vi "simula cmecc.vi"(0 "RPM":dbl format="%#_13g", 1 "C":dbl format="%#_13g", 2 "String":string="CARICO", 3 "V":dbl format="%#_13g") -> (12 "RPM":dbl, 14 "cosfi":dbl, 15 "C[nm]":dbl, 16 "I[A]":dbl, 17 "Pin kw":dbl, 18 "Pout kw":dbl, 19 "eff%":dbl)   [LabVIEW 2019]
uses:
  <vilib>/gmath/NI_Gmath.lvlib
panel:
  in  "VUOTO":string[][](array[string])=[["n°Acq", "Freq [Hz]", "RPM", "Vtr [V]", "Vts [V]", "Vsr [V]", "It [A]", "Ir [A]", "Is [A]", "Vmean [V]", "Imean [A]", "Irec [A]", "Irec/In", "CosFi", "P in [kW]", "P out [kW]", "Eff [%]", "T [Nm]", "Trec [Nm]", "Trec/Cn", "Slip [%]", "R1 [Ohm]", "dT1 [°C]", "Tamb [°C]", "TC1 [°C]", "TC2 [°C]", "TC3 [°C]", "Time [min]", "Date\\time"], ["1", "49.99", "2990", "441.34", "414.63", "442.09", "1.90", "1.98", "2.04", "441.72", "1.97", "1.78", "0.76", "0.125", "0.189", "0.000", "0.00", "0.01", "0.01", "0.00", "100.00", "14.20449", "0.79", "21.8", "32.9", "30.7", "28.8", "1.373", "24/05/2017 16:33:41"], ["2", "50.00", "2990", "399.24", "374.56", "401.38", "1.14", "1.25", "1.30", "400.31", "1.22", "1.22", "0.52", "0.142", "0.121", "0.000", "0.00", "0.01", "0.01", "0.00", "100.00", "14.24889", "1.58", "21.9", "32.5", "29.7", "28.2", "1.890", "24/05/2017 16:34:12"], ["3", "50.01", "2990", "377.89", "353.26", "380.50", "0.90", "1.02", "1.07", "379.20", "0.99", "1.04", "0.44", "0.161", "0.104", "0.000", "0.00", "0.01", "0.01", "0.00", "100.00", "14.19922", "0.69", "21.8", "32.1", "29.2", "27.9", "2.373", "24/05/2017 16:34:41"], ["4", "50.02", "2990", "359.59", "333.88", "361.83", "0.77", "0.89", "0.91", "360.71", "0.84", "0.93", "0.39", "0.182", "0.095", "0.000", "0.00", "0.01", "0.01", "0.00", "100.00", "14.12952", "-0.59", "21.9", "31.9", "28.8", "27.7", "2.866", "24/05/2017 16:35:11"], ["5", "49.98", "2990", "239.37", "220.27", "242.66", "0.39", "0.51", "0.52", "241.01", "0.46", "0.76", "0.32", "0.340", "0.065", "0.000", "0.00", "0.01", "0.02", "0.00", "100.00", "14.03546", "-2.31", "21.9", "31.5", "28.6", "27.5", "3.440", "24/05/2017 16:35:45"], ["6", "49.99", "2990", "199.14", "180.73", "202.29", "0.33", "0.44", "0.44", "200.72", "0.38", "0.76", "0.32", "0.440", "0.059", "0.000", "0.00", "0.01", "0.02", "0.01", "100.00", "13.96122", "-3.66", "21.9", "31.3", "28.4", "27.4", "3.890", "24/05/2017 16:36:12"], ["7", "49.99", "2990", "159.38", "140.24", "162.50", "0.27", "0.41", "0.37", "160.94", "0.32", "0.81", "0.34", "0.599", "0.054", "0.000", "0.00", "0.01", "0.04", "0.01", "100.00", "13.90466", "-4.68", "21.9", "31.0", "28.2", "27.2", "4.256", "24/05/2017 16:36:34"], ["8", "49.99", "2990", "120.04", "101.13", "122.43", "0.28", "0.38", "0.34", "121.23", "0.31", "1.03", "0.43", "0.790", "0.052", "0.000", "0.00", "0.01", "0.06", "0.02", "100.00", "13.84049", "-5.84", "21.9", "30.7", "27.9", "27.0", "4.703", "24/05/2017 16:37:01"]]
  in  "CARICO":string[][](array[string])=[["n°Acq", "Freq [Hz]", "RPM", "Vtr [V]", "Vts [V]", "Vsr [V]", "It [A]", "Ir [A]", "Is [A]", "Vmean [V]", "Imean [A]", "Irec [A]", "Irec/In", "CosFi", "P in [kW]", "P out [kW]", "Eff [%]", "T [Nm]", "Trec [Nm]", "Trec/Cn", "Slip [%]", "R1 [Ohm]", "dT1 [°C]", "Tamb [°C]", "TC1 [°C]", "TC2 [°C]", "TC3 [°C]", "Time [min]", "Date\\time"], ["1", "50.01", "2806.2", "400.30", "376.15", "401.45", "2.86", "2.99", "2.95", "400.87", "2.90", "2.89", "1.23", "0.880", "1.771", "1.372", "77.48", "4.67", "4.65", "1.27", "6.47", "14.78061", "8.97", "21.9", "33.2", "30.2", "28.9", "1.737", "24/05/2017 16:26:19"], ["2", "50.00", "2828.6", "400.27", "376.11", "401.72", "2.57", "2.72", "2.67", "400.99", "2.62", "2.62", "1.11", "0.870", "1.585", "1.246", "78.58", "4.21", "4.18", "1.15", "5.71", "15.05714", "13.92", "21.9", "33.0", "29.6", "28.6", "2.673", "24/05/2017 16:27:15"], ["3", "50.00", "2863.3", "399.24", "375.18", "400.70", "2.18", "2.32", "2.28", "399.97", "2.23", "2.23", "0.95", "0.843", "1.303", "1.043", "80.03", "3.48", "3.48", "0.95", "4.56", "15.05270", "13.85", "21.9", "32.9", "29.3", "28.6", "3.903", "24/05/2017 16:28:29"], ["4", "49.99", "2898.6", "398.36", "374.57", "400.21", "1.78", "1.93", "1.89", "399.29", "1.84", "1.84", "0.78", "0.788", "1.002", "0.808", "80.72", "2.66", "2.67", "0.73", "3.36", "14.99414", "12.80", "21.9", "32.9", "29.4", "28.5", "4.370", "24/05/2017 16:28:57"], ["5", "50.00", "2935.4", "397.64", "373.91", "399.71", "1.41", "1.56", "1.55", "398.67", "1.48", "1.48", "0.63", "0.667", "0.681", "0.535", "78.58", "1.74", "1.75", "0.48", "2.15", "14.88601", "10.84", "21.9", "32.8", "29.2", "28.4", "4.823", "24/05/2017 16:29:24"], ["6", "50.00", "2967.6", "398.04", "373.91", "400.09", "1.18", "1.33", "1.33", "399.06", "1.26", "1.26", "0.53", "0.446", "0.388", "0.267", "68.91", "0.86", "0.86", "0.24", "1.08", "14.75175", "8.44", "21.9", "32.8", "29.2", "28.3", "5.307", "24/05/2017 16:29:53"]]
  in  "CMECC":string[][](array[string])=[["n°Acq", "Freq [Hz]", "RPM", "Vtr [V]", "Vts [V]", "Vsr [V]", "It [A]", "Ir [A]", "Is [A]", "Vmean [V]", "Imean [A]", "Irec [A]", "Irec/In", "CosFi", "P in [kW]", "P out [kW]", "Eff [%]", "T [Nm]", "Trec [Nm]", "Trec/Cn", "Slip [%]", "R1 [Ohm]", "dT1 [°C]", "Tamb [°C]", "TC1 [°C]", "TC2 [°C]", "TC3 [°C]", "Time [min]", "Date\\time", "", "", "", ""], ["0", "49,8", "3010", "400", "377", "400", "0,8", "0,4", "0,7", "400", "0,85", "", "", "", "0,3", "0", "", "0", "", "", "", "", "", "", "", "", "", "", "", "", "", "", ""], ["1", "49.98", "2948.1", "399.34", "377.38", "401.04", "1.36", "1.49", "1.48", "400.19", "1.42", "1.42", "0.60", "0.608", "0.599", "0.455", "75.96", "1.47", "1.47", "0.40", "1.69", "-1.00000", "0.00", "22.3", "30.3", "28.4", "27.3", "0.977", "25/05/2017 14:23:00", "", "", "", ""], ["2", "49.98", "2902.9", "398.17", "375.99", "399.91", "1.72", "1.85", "1.82", "399.04", "1.77", "1.77", "0.75", "0.766", "0.937", "0.810", "86.44", "2.66", "2.68", "0.73", "3.20", "-1.00000", "0.00", "22.3", "30.3", "28.4", "27.3", "0.989", "25/05/2017 14:23:00", "", "", "", ""], ["3", "49.98", "2853.7", "397.65", "376.18", "399.71", "2.30", "2.47", "2.43", "398.68", "2.37", "2.37", "1.01", "0.854", "1.396", "1.153", "82.60", "3.86", "3.88", "1.06", "4.84", "-1.00000", "0.00", "22.3", "30.3", "28.4", "27.3", "1.001", "25/05/2017 14:23:01", "", "", "", ""], ["4", "49.99", "2803.6", "396.44", "374.24", "398.18", "2.88", "3.01", "3.00", "397.31", "2.94", "2.96", "1.25", "0.882", "1.784", "1.427", "79.99", "4.86", "4.93", "1.35", "6.52", "-1.00000", "0.00", "22.3", "30.2", "28.4", "27.2", "1.014", "25/05/2017 14:23:02", "", "", "", ""], ["5", "49.99", "2759.2", "397.71", "375.43", "399.21", "3.46", "3.58", "3.56", "398.46", "3.51", "3.52", "1.49", "0.891", "2.157", "1.644", "76.22", "5.69", "5.73", "1.57", "8.01", "-1.00000", "0.00", "22.3", "30.2", "28.4", "27.2", "1.027", "25/05/2017 14:23:03", "", "", "", ""], ["6", "49.99", "2710.3", "395.68", "373.27", "397.27", "3.98", "4.10", "4.08", "396.47", "4.03", "4.07", "1.72", "0.895", "2.479", "1.807", "72.88", "6.37", "6.48", "1.78", "9.64", "-1.00000", "0.00", "22.3", "30.2", "28.4", "27.2", "1.040", "25/05/2017 14:23:03", "", "", "", ""], ["7", "49.92", "2666.1", "396.88", "375.28", "398.43", "4.44", "4.54", "4.54", "397.66", "4.49", "4.51", "1.91", "0.894", "2.765", "1.942", "70.23", "6.96", "7.04", "1.93", "10.99", "-1.00000", "0.00", "22.3", "30.2", "28.3", "27.2", "1.052", "25/05/2017 14:23:04", "", "", "", ""], ["8", "49.99", "2623.2", "395.30", "373.16", "396.73", "4.85", "4.93", "4.94", "396.01", "4.89", "4.94", "2.09", "0.894", "3.001", "2.029", "67.61", "7.39", "7.54", "2.06", "12.54", "-1.00000", "0.00", "22.3", "30.2", "28.3", "27.2", "1.062", "25/05/2017 14:23:05", "", "", "", ""], ["9", "49.99", "2560.8", "394.56", "372.80", "396.07", "5.43", "5.52", "5.52", "395.31", "5.47", "5.54", "2.35", "0.892", "3.344", "2.184", "65.30", "8.14", "8.34", "2.28", "14.63", "-1.00000", "0.00", "22.3", "30.2", "28.3", "27.2", "1.073", "25/05/2017 14:23:05", "", "", "", ""], ["10", "49.99", "2490.5", "400.92", "378.49", "402.07", "6.10", "6.19", "6.16", "401.50", "6.13", "6.11", "2.59", "0.888", "3.787", "2.319", "61.25", "8.89", "8.83", "2.42", "16.96", "-1.00000", "0.00", "22.3", "30.2", "28.3", "27.2", "1.083", "25/05/2017 14:23:06", "", "", "", ""], ["11", "49.99", "2409.2", "400.46", "378.67", "402.05", "6.79", "6.88", "6.88", "401.25", "6.84", "6.81", "2.89", "0.884", "4.199", "2.342", "55.79", "9.28", "9.23", "2.53", "19.68", "-1.00000", "0.00", "22.3", "30.2", "28.3", "27.2", "1.093", "25/05/2017 14:23:07", "", "", "", ""], ["12", "49.99", "2338.6", "400.74", "377.60", "402.36", "7.33", "7.43", "7.42", "401.55", "7.37", "7.35", "3.11", "0.879", "4.508", "2.357", "52.29", "9.63", "9.55", "2.62", "22.03", "-1.00000", "0.00", "22.3", "30.2", "28.3", "27.2", "1.103", "25/05/2017 14:23:07", "", "", "", ""], ["13", "49.98", "2266.1", "400.56", "376.81", "401.95", "7.83", "7.93", "7.90", "401.25", "7.87", "7.84", "3.32", "0.874", "4.781", "2.338", "48.91", "9.85", "9.79", "2.68", "24.44", "-1.00000", "0.00", "22.3", "30.2", "28.3", "27.2", "1.113", "25/05/2017 14:23:08", "", "", "", ""], ["14", "50.00", "2194.0", "400.26", "377.09", "401.37", "8.28", "8.38", "8.35", "400.82", "8.31", "8.29", "3.51", "0.870", "5.018", "2.298", "45.79", "10.00", "9.96", "2.73", "26.87", "-1.00000", "0.00", "22.3", "30.2", "28.3", "27.2", "1.124", "25/05/2017 14:23:08", "", "", "", ""], ["15", "50.00", "2126.8", "399.39", "376.25", "401.11", "8.66", "8.76", "8.73", "400.25", "8.69", "8.69", "3.68", "0.866", "5.217", "2.245", "43.03", "10.08", "10.07", "2.76", "29.10", "-1.00000", "0.00", "22.3", "30.2", "28.3", "27.2", "1.134", "25/05/2017 14:23:09", "", "", "", ""], ["16", "49.99", "2052.7", "401.77", "378.90", "403.07", "9.02", "9.14", "9.10", "402.42", "9.06", "9.01", "3.82", "0.863", "5.449", "2.181", "40.02", "10.15", "10.02", "2.75", "31.56", "-1.00000", "0.00", "22.3", "30.2", "28.3", "27.2", "1.144", "25/05/2017 14:23:10", "", "", "", ""], ["17", "49.98", "1980.2", "397.93", "375.13", "399.39", "9.34", "9.45", "9.40", "398.66", "9.37", "9.41", "3.99", "0.858", "5.553", "2.075", "37.36", "10.00", "10.07", "2.76", "33.97", "-1.00000", "0.00", "22.3", "30.3", "28.3", "27.2", "1.154", "25/05/2017 14:23:10", "", "", "", ""], ["18", "49.98", "1916.4", "398.56", "374.54", "399.91", "9.63", "9.74", "9.70", "399.23", "9.67", "9.69", "4.10", "0.855", "5.713", "2.026", "35.46", "10.09", "10.13", "2.78", "36.09", "-1.00000", "0.00", "22.3", "30.3", "28.3", "27.2", "1.164", "25/05/2017 14:23:11", "", "", "", ""], ["19", "49.99", "1844.1", "398.95", "376.55", "400.02", "9.91", "10.04", "10.00", "399.48", "9.96", "9.97", "4.22", "0.851", "5.865", "1.925", "32.83", "9.97", "10.00", "2.74", "38.51", "-1.00000", "0.00", "22.3", "30.3", "28.3", "27.2", "1.174", "25/05/2017 14:23:11", "", "", "", ""], ["20", "49.98", "1771.5", "397.82", "375.33", "398.67", "10.15", "10.27", "10.21", "398.25", "10.18", "10.22", "4.33", "0.848", "5.955", "1.814", "30.46", "9.78", "9.86", "2.70", "40.93", "-1.00000", "0.00", "22.2", "30.3", "28.3", "27.3", "1.185", "25/05/2017 14:23:12", "", "", "", ""], ["21", "49.98", "1706.2", "397.07", "374.33", "397.98", "10.37", "10.46", "10.40", "397.53", "10.39", "10.45", "4.43", "0.845", "6.044", "1.733", "28.68", "9.70", "9.82", "2.69", "43.11", "-1.00000", "0.00", "22.2", "30.3", "28.3", "27.3", "1.195", "25/05/2017 14:23:13", "", "", "", ""], ["22", "49.99", "1634.2", "397.30", "374.02", "398.72", "10.57", "10.68", "10.64", "398.01", "10.61", "10.66", "4.52", "0.843", "6.163", "1.652", "26.80", "9.65", "9.75", "2.67", "45.52", "-1.00000", "0.00", "22.2", "30.3", "28.3", "27.3", "1.205", "25/05/2017 14:23:13", "", "", "", ""], ["23", "49.99", "1552.9", "396.22", "373.07", "397.11", "10.79", "10.88", "10.85", "396.67", "10.82", "10.91", "4.62", "0.839", "6.236", "1.530", "24.53", "9.41", "9.57", "2.62", "48.23", "-1.00000", "0.00", "22.2", "30.3", "28.3", "27.3", "1.215", "25/05/2017 14:23:14", "", "", "", ""], ["24", "49.99", "1478.5", "398.04", "375.15", "398.88", "11.02", "11.12", "11.05", "398.46", "11.04", "11.08", "4.69", "0.838", "6.378", "1.443", "22.62", "9.32", "9.39", "2.57", "50.70", "-1.00000", "0.00", "22.3", "30.5", "28.3", "27.4", "1.225", "25/05/2017 14:23:14", "", "", "", ""], ["25", "49.98", "1409.6", "396.79", "373.74", "398.12", "11.15", "11.25", "11.21", "397.46", "11.18", "11.26", "4.77", "0.835", "6.431", "1.350", "20.99", "9.14", "9.26", "2.54", "53.00", "-1.00000", "0.00", "22.3", "30.5", "28.3", "27.4", "1.235", "25/05/2017 14:23:15", "", "", "", ""], ["26", "49.98", "1346.7", "396.48", "373.50", "397.29", "11.28", "11.39", "11.34", "396.89", "11.31", "11.40", "4.83", "0.833", "6.474", "1.263", "19.50", "8.95", "9.09", "2.49", "55.09", "-1.00000", "0.00", "22.3", "30.5", "28.3", "27.4", "1.246", "25/05/2017 14:23:16", "", "", "", ""], ["27", "49.99", "1265.5", "396.37", "373.49", "396.93", "11.37", "11.48", "11.41", "396.65", "11.39", "11.49", "4.87", "0.832", "6.510", "1.151", "17.69", "8.69", "8.84", "2.42", "57.81", "-1.00000", "0.00", "22.3", "30.6", "28.3", "27.5", "1.256", "25/05/2017 14:23:16", "", "", "", ""], ["28", "49.98", "1212.3", "400.93", "377.63", "401.91", "11.64", "11.72", "11.68", "401.42", "11.66", "11.62", "4.92", "0.832", "6.741", "1.138", "16.89", "8.97", "8.90", "2.44", "59.57", "-1.00000", "0.00", "22.3", "30.6", "28.3", "27.5", "1.266", "25/05/2017 14:23:17", "", "", "", ""], ["29", "49.99", "1137.2", "403.35", "380.25", "404.47", "11.91", "11.98", "11.88", "403.91", "11.90", "11.78", "4.99", "0.830", "6.908", "1.062", "15.37", "8.92", "8.75", "2.40", "62.08", "-1.00000", "0.00", "22.3", "30.6", "28.3", "27.5", "1.276", "25/05/2017 14:23:18", "", "", "", ""], ["30", "49.98", "1058.9", "402.43", "378.57", "403.46", "11.93", "12.03", "12.00", "402.94", "11.97", "11.88", "5.03", "0.829", "6.923", "0.946", "13.66", "8.53", "8.40", "2.30", "64.69", "-1.00000", "0.00", "22.3", "30.6", "28.3", "27.5", "1.286", "25/05/2017 14:23:18", "", "", "", ""], ["31", "49.97", "986.7", "401.35", "378.20", "402.45", "12.00", "12.07", "12.05", "401.90", "12.03", "11.97", "5.07", "0.827", "6.928", "0.859", "12.40", "8.31", "8.24", "2.26", "67.09", "-1.00000", "0.00", "22.3", "30.7", "28.4", "27.6", "1.297", "25/05/2017 14:23:19", "", "", "", ""], ["32", "49.99", "920.0", "402.00", "378.51", "403.04", "12.08", "12.17", "12.13", "402.52", "12.11", "12.03", "5.10", "0.827", "6.975", "0.791", "11.34", "8.21", "8.11", "2.22", "69.33", "-1.00000", "0.00", "22.3", "30.7", "28.4", "27.6", "1.307", "25/05/2017 14:23:19", "", "", "", ""], ["33", "49.98", "850.8", "401.64", "378.11", "402.78", "12.17", "12.25", "12.22", "402.21", "12.19", "12.13", "5.14", "0.826", "7.013", "0.705", "10.06", "7.92", "7.83", "2.14", "71.63", "-1.00000", "0.00", "22.3", "30.7", "28.4", "27.6", "1.317", "25/05/2017 14:23:20", "", "", "", ""], ["34", "49.97", "777.8", "400.86", "378.12", "402.49", "12.19", "12.27", "12.23", "401.67", "12.21", "12.16", "5.15", "0.825", "7.007", "0.640", "9.13", "7.85", "7.79", "2.13", "74.06", "-1.00000", "0.00", "22.3", "30.9", "28.5", "27.8", "1.327", "25/05/2017 14:23:21", "", "", "", ""], ["35", "49.97", "705.5", "400.85", "378.16", "403.38", "12.26", "12.37", "12.34", "402.12", "12.30", "12.23", "5.18", "0.825", "7.069", "0.562", "7.96", "7.61", "7.53", "2.06", "76.47", "-1.00000", "0.00", "22.3", "30.9", "28.5", "27.8", "1.337", "25/05/2017 14:23:21", "", "", "", ""], ["36", "49.98", "637.0", "401.49", "378.85", "403.76", "12.34", "12.45", "12.41", "402.62", "12.37", "12.29", "5.21", "0.824", "7.112", "0.490", "6.88", "7.34", "7.24", "1.98", "78.76", "-1.00000", "0.00", "22.3", "30.9", "28.5", "27.8", "1.347", "25/05/2017 14:23:22", "", "", "", ""], ["37", "49.99", "578.9", "401.68", "378.71", "403.39", "12.34", "12.46", "12.42", "402.53", "12.38", "12.30", "5.21", "0.824", "7.109", "0.443", "6.23", "7.30", "7.21", "1.98", "80.70", "-1.00000", "0.00", "22.3", "30.9", "28.5", "27.8", "1.358", "25/05/2017 14:23:22", "", "", "", ""], ["38", "49.98", "489.3", "399.20", "375.75", "400.56", "12.30", "12.39", "12.34", "399.88", "12.32", "12.32", "5.22", "0.822", "7.009", "0.359", "5.13", "7.01", "7.02", "1.92", "83.69", "-1.00000", "0.00", "22.3", "31.0", "28.7", "28.0", "1.368", "25/05/2017 14:23:23", "", "", "", ""], ["39", "49.98", "436.2", "396.67", "374.25", "397.73", "12.21", "12.28", "12.26", "397.20", "12.24", "12.33", "5.22", "0.822", "6.921", "0.315", "4.55", "6.90", "7.00", "1.92", "85.45", "-1.00000", "0.00", "22.3", "31.0", "28.7", "28.0", "1.378", "25/05/2017 14:23:24", "", "", "", ""], ["40", "50.02", "372.9", "398.90", "376.64", "399.52", "12.35", "12.37", "12.31", "399.21", "12.33", "12.35", "5.23", "0.823", "7.013", "0.274", "3.91", "7.02", "7.04", "1.93", "87.58", "-1.00000", "0.00", "22.3", "31.0", "28.7", "28.0", "1.388", "25/05/2017 14:23:24", "", "", "", ""], ["41", "49.99", "298.8", "399.29", "376.66", "399.94", "12.33", "12.41", "12.37", "399.62", "12.35", "12.36", "5.24", "0.821", "7.018", "0.222", "3.16", "7.09", "7.10", "1.95", "90.04", "-1.00000", "0.00", "22.3", "31.0", "28.7", "28.0", "1.399", "25/05/2017 14:23:25", "", "", "", ""], ["42", "49.97", "230.7", "398.30", "375.72", "399.25", "12.32", "12.37", "12.36", "398.78", "12.34", "12.38", "5.24", "0.821", "7.001", "0.173", "2.47", "7.15", "7.19", "1.97", "92.30", "-1.00000", "0.00", "22.3", "31.3", "28.8", "28.3", "1.409", "25/05/2017 14:23:25", "", "", "", ""], ["43", "49.98", "187.8", "399.13", "376.39", "399.68", "12.31", "12.37", "12.36", "399.41", "12.34", "12.35", "5.23", "0.822", "7.011", "0.152", "2.17", "7.75", "7.77", "2.13", "93.74", "-1.00000", "0.00", "22.3", "31.3", "28.8", "28.3", "1.419", "25/05/2017 14:23:26", "", "", "", ""], ["44", "50.00", "83.9", "399.74", "376.53", "400.38", "12.32", "12.37", "12.40", "400.06", "12.36", "12.36", "5.24", "0.823", "7.053", "0.069", "0.98", "7.88", "7.88", "2.16", "97.20", "-1.00000", "0.00", "22.3", "31.3", "28.8", "28.3", "1.429", "25/05/2017 14:23:27", "", "", "", ""], ["45", "49.97", "3,2", "399.16", "376.52", "400.07", "12.35", "12.43", "12.35", "399.62", "12.35", "12.36", "5.24", "0.824", "7.046", "0.003", "0.04", "7.87", "7.88", "2.16", "99.87", "-1.00000", "0.00", "22.3", "31.4", "29.0", "28.5", "1.440", "25/05/2017 14:23:27", "", "", "", ""]]
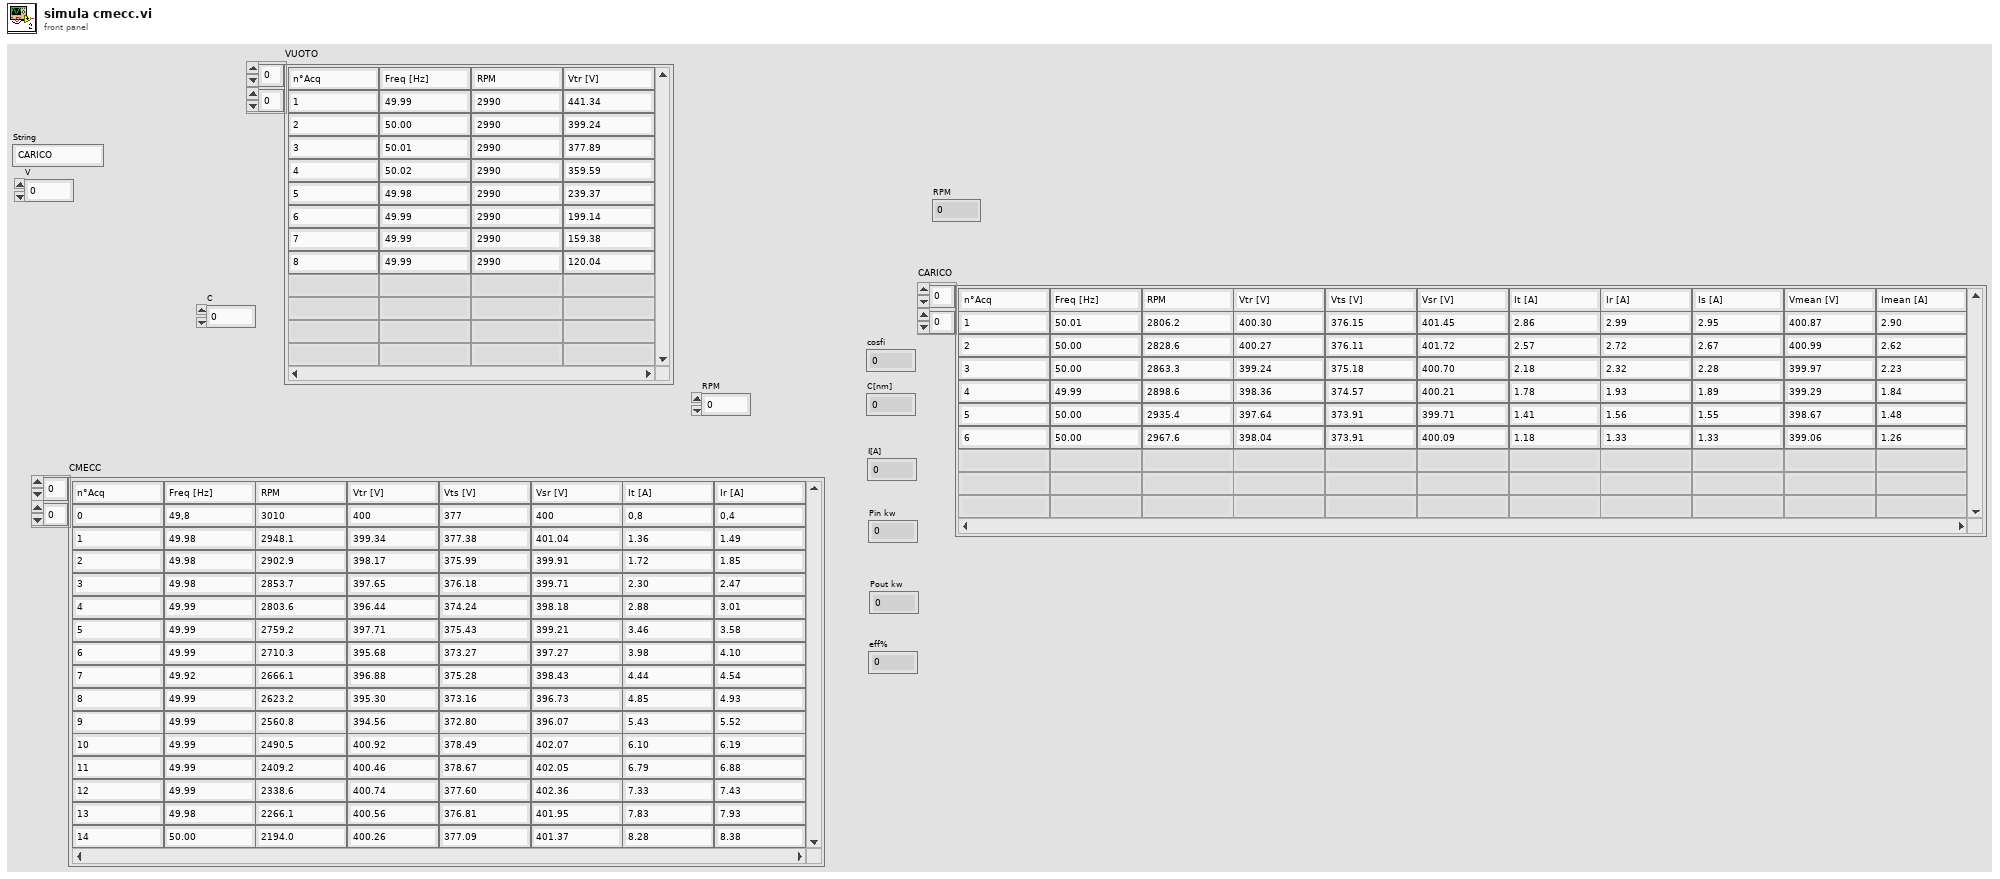
[diagram p1: front panel]
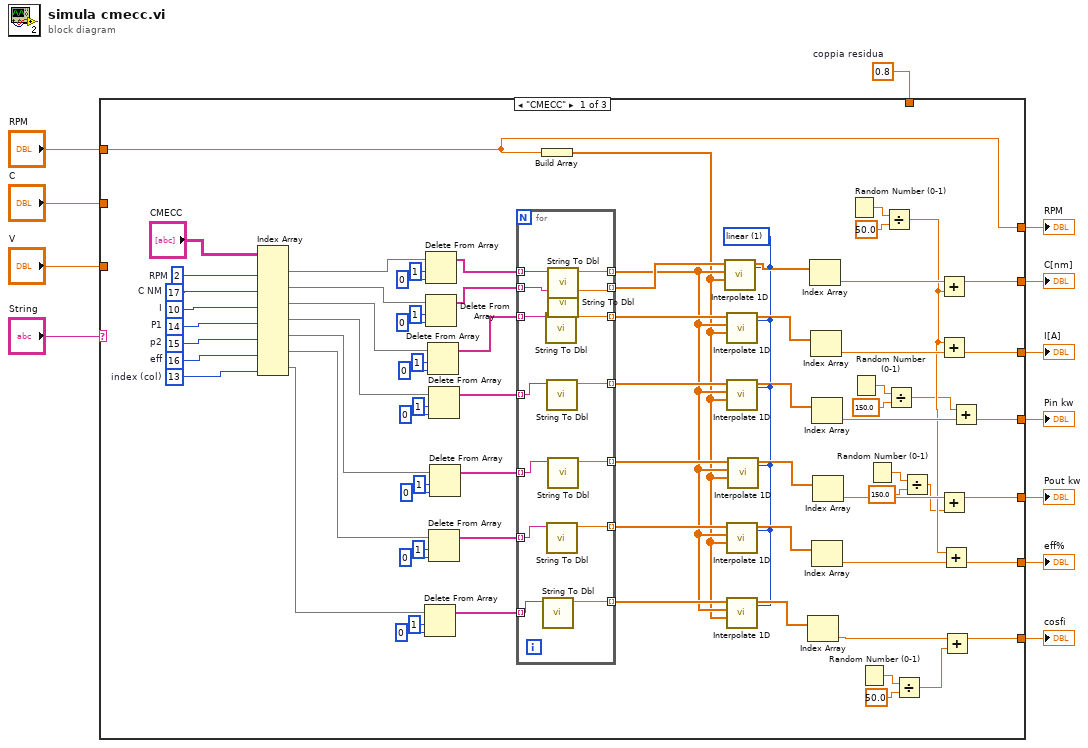
[diagram p0: block diagram]
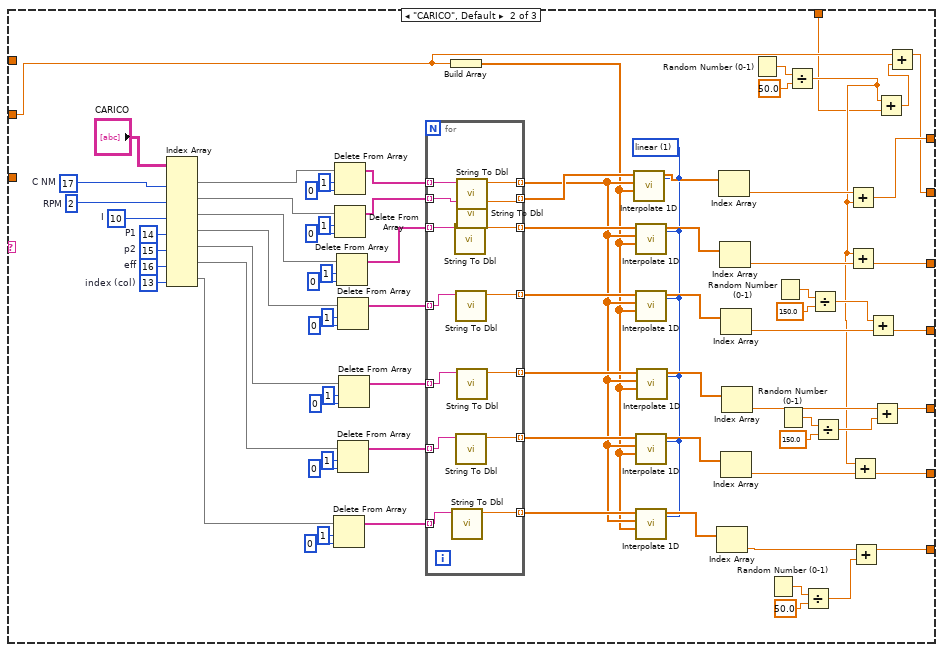
[diagram p2: hidden frame]
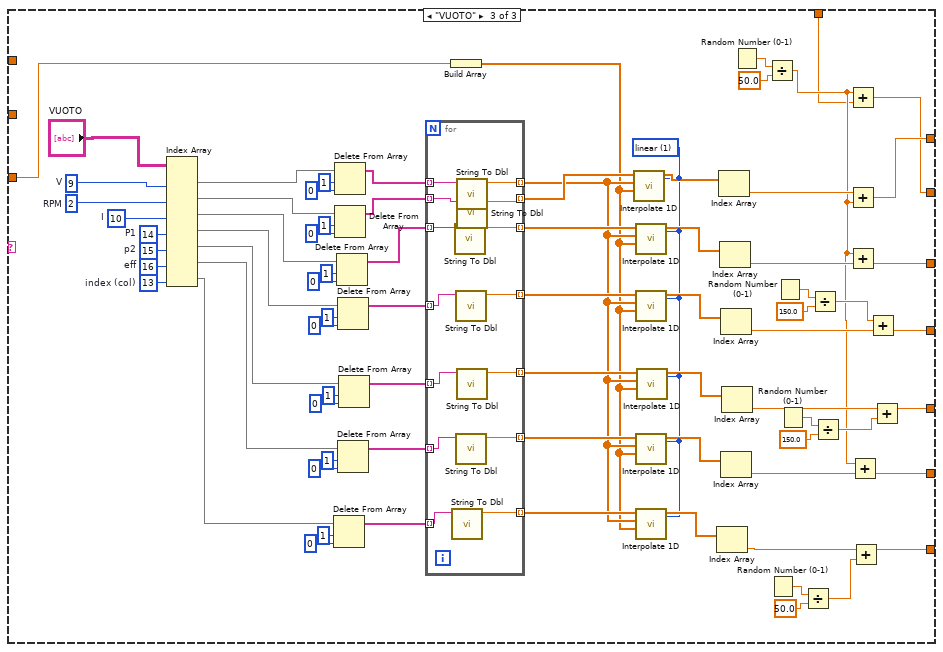
[diagram p3: hidden frame]
diagram:
  w1 = 0.8  # coppia residua
  n1 = case shown="\"CMECC\"" "String" {
    tunnel: [w29 w105 w196] -> w12
    tunnel: [w28 w127 w219] -> w11
    tunnel: [w27 w126 w218] -> w10
    tunnel: [w26 w125 w217] -> w9
    tunnel: [w25 w124 w216] -> w8
    tunnel: [w24 w123 w215] -> w7
    tunnel: "RPM" -> [w19 _ _]
    tunnel: "C" -> [_ w115 _]
    tunnel: [w19 w116 w209] -> w3
    tunnel: "V" -> [_ _ w201]
    tunnel: w1 -> [_ w103 w197]
    frame "CMECC" {
      w42 = 13  # index (col)
      w50 = 16  # eff
      w52 = 15  # p2
      w59 = 14  # P1
      w72 = 10  # I
      w32 = 1 items=["nearest", "linear", "spline", "cubic Hermite", "Lagrange"] ("method")
      w83 = 17  # C NM
      w87 = 2  # RPM
      n2 = Index Array(array="CMECC", index (col) #1=w87, index (col) #2=w83, index (col) #3=w72, index (col) #4=w59, index (col) #5=w52, index (col) #6=w50, index (col) #7=w42) -> (element #1=w82:string[], element #2=w76:string[], element #3=w71:string[], element #4=w61:string[], element #5=w51:string[], element #6=w43:string[], element #7=w36:string[])  [unwired: 7 in]
      n3 = Delete From Array(array=w36, length=1, index=0) -> (array with subset deleted=w41:string[])  [unwired: 1 out]
      n4 = Delete From Array(array=w82, length=1, index=0) -> (array with subset deleted=w81:string[])  [unwired: 1 out]
      n5 = Delete From Array(array=w76, length=1, index=0) -> (array with subset deleted=w75:string[])  [unwired: 1 out]
      n6 = Delete From Array(array=w71, length=1, index=0) -> (array with subset deleted=w70:string[])  [unwired: 1 out]
      n7 = Delete From Array(array=w61, length=1, index=0) -> (array with subset deleted=w60:string[])  [unwired: 1 out]
      n8 = Delete From Array(array=w43, length=1, index=0) -> (array with subset deleted=w44:string[])  [unwired: 1 out]
      n9 = Delete From Array(array=w51, length=1, index=0) -> (array with subset deleted=w58:string[])  [unwired: 1 out]
      n10 = for {
        tunnel: w81 -> [w102] mode=indexing
        tunnel: [w101] -> w34 mode=indexing
        tunnel: w75 -> [w100] mode=indexing
        tunnel: [w99] -> w86 mode=indexing
        tunnel: w70 -> [w98] mode=indexing
        tunnel: [w97] -> w69 mode=indexing
        tunnel: [w96] -> w64 mode=indexing
        tunnel: w60 -> [w95] mode=indexing
        tunnel: [w93] -> w55 mode=indexing
        tunnel: w58 -> [w94] mode=indexing
        tunnel: [w92] -> w47 mode=indexing
        tunnel: w44 -> [w91] mode=indexing
        tunnel: [w89] -> w38 mode=indexing
        tunnel: w41 -> [w90] mode=indexing
        n11 = call "String To Dbl.vi"("String"=w90) -> ("Numeric"=w89:dbl)  [unwired: 10 in]
        n12 = call "String To Dbl.vi"("String"=w98) -> ("Numeric"=w97:dbl)  [unwired: 10 in]
        n13 = call "String To Dbl.vi"("String"=w95) -> ("Numeric"=w96:dbl)  [unwired: 10 in]
        n14 = call "String To Dbl.vi"("String"=w91) -> ("Numeric"=w92:dbl)  [unwired: 10 in]
        n15 = call "String To Dbl.vi"("String"=w102) -> ("Numeric"=w101:dbl)  [unwired: 10 in]
        n16 = call "String To Dbl.vi"("String"=w100) -> ("Numeric"=w99:dbl)  [unwired: 10 in]
        n17 = call "String To Dbl.vi"("String"=w94) -> ("Numeric"=w93:dbl)  [unwired: 10 in]
      }
      n18 = Build Array(w19) -> (w33:dbl[])
      n19 = call <vilib>:"Interpolate 1D.vi"("method"=w32, "xi"=w33, "X"=w34, "Y"=w86) -> ("yi"=w85:dbl[])  [unwired: 5 in, 2 out]
      n20 = call <vilib>:"Interpolate 1D.vi"("method"=w32, "xi"=w33, "X"=w34, "Y"=w69) -> ("yi"=w67:dbl[])  [unwired: 5 in, 2 out]
      n21 = call <vilib>:"Interpolate 1D.vi"("method"=w32, "xi"=w33, "X"=w34, "Y"=w64) -> ("yi"=w66:dbl[])  [unwired: 5 in, 2 out]
      n22 = call <vilib>:"Interpolate 1D.vi"("method"=w32, "xi"=w33, "X"=w34, "Y"=w47) -> ("yi"=w49:dbl[])  [unwired: 5 in, 2 out]
      n23 = call <vilib>:"Interpolate 1D.vi"("method"=w32, "xi"=w33, "X"=w34, "Y"=w38) -> ("yi"=w37:dbl[])  [unwired: 5 in, 2 out]
      n24 = call <vilib>:"Interpolate 1D.vi"("method"=w32, "xi"=w33, "X"=w34, "Y"=w55) -> ("yi"=w53:dbl[])  [unwired: 5 in, 2 out]
      n25 = Index Array(array=w37) -> (element=w35:dbl)  [unwired: 1 in]
      n26 = Index Array(array=w85) -> (element=w84:dbl)  [unwired: 1 in]
      n27 = Index Array(array=w67) -> (element=w68:dbl)  [unwired: 1 in]
      n28 = Index Array(array=w66) -> (element=w65:dbl)  [unwired: 1 in]
      n29 = Index Array(array=w49) -> (element=w48:dbl)  [unwired: 1 in]
      n30 = Index Array(array=w53) -> (element=w54:dbl)  [unwired: 1 in]
      n31 = Random Number (0-1)() -> (number: 0 to 1=w31:dbl)
      n32 = Random Number (0-1)() -> (number: 0 to 1=w17:dbl)
      n33 = Random Number (0-1)() -> (number: 0 to 1=w21:dbl)
      n34 = Random Number (0-1)() -> (number: 0 to 1=w15:dbl)
      n35 = Divide(x=w31, y=50.0) -> (x/y=w23:dbl)
      n36 = Divide(x=w17, y=150.0) -> (x/y=w16:dbl)
      n37 = Divide(x=w21, y=50.0) -> (x/y=w20:dbl)
      n38 = Divide(x=w15, y=150.0) -> (x/y=w13:dbl)
      n39 = Add(x=w84, y=w23) -> (x+y=w29:dbl)
      n40 = Add(x=w23, y=w68) -> (x+y=w28:dbl)
      n41 = Add(x=w54, y=w13) -> (x+y=w26:dbl)
      n42 = Add(x=w23, y=w48) -> (x+y=w25:dbl)
      n43 = Add(x=w35, y=w20) -> (x+y=w24:dbl)
      n44 = Add(x=w16, y=w65) -> (x+y=w27:dbl)
    }
    frame "CARICO", Default {
      w138 = 13  # index (col)
      w146 = 16  # eff
      w148 = 15  # p2
      w155 = 14  # P1
      w168 = 10  # I
      w128 = 1 items=["nearest", "linear", "spline", "cubic Hermite", "Lagrange"] ("method")
      w118 = 17  # C NM
      w117 = 2  # RPM
      n45 = Index Array(array="CARICO", index (col) #1=w118, index (col) #2=w117, index (col) #3=w168, index (col) #4=w155, index (col) #5=w148, index (col) #6=w146, index (col) #7=w138) -> (element #1=w178:string[], element #2=w172:string[], element #3=w167:string[], element #4=w157:string[], element #5=w147:string[], element #6=w139:string[], element #7=w132:string[])  [unwired: 7 in]
      n46 = Delete From Array(array=w132, length=1, index=0) -> (array with subset deleted=w137:string[])  [unwired: 1 out]
      n47 = Delete From Array(array=w178, length=1, index=0) -> (array with subset deleted=w177:string[])  [unwired: 1 out]
      n48 = Delete From Array(array=w172, length=1, index=0) -> (array with subset deleted=w171:string[])  [unwired: 1 out]
      n49 = Delete From Array(array=w167, length=1, index=0) -> (array with subset deleted=w166:string[])  [unwired: 1 out]
      n50 = Delete From Array(array=w157, length=1, index=0) -> (array with subset deleted=w156:string[])  [unwired: 1 out]
      n51 = Delete From Array(array=w139, length=1, index=0) -> (array with subset deleted=w140:string[])  [unwired: 1 out]
      n52 = Delete From Array(array=w147, length=1, index=0) -> (array with subset deleted=w154:string[])  [unwired: 1 out]
      n53 = for {
        tunnel: w177 -> [w195] mode=indexing
        tunnel: [w194] -> w130 mode=indexing
        tunnel: w171 -> [w193] mode=indexing
        tunnel: [w192] -> w181 mode=indexing
        tunnel: w166 -> [w191] mode=indexing
        tunnel: [w190] -> w165 mode=indexing
        tunnel: [w189] -> w160 mode=indexing
        tunnel: w156 -> [w188] mode=indexing
        tunnel: [w186] -> w151 mode=indexing
        tunnel: w154 -> [w187] mode=indexing
        tunnel: [w185] -> w143 mode=indexing
        tunnel: w140 -> [w184] mode=indexing
        tunnel: [w182] -> w134 mode=indexing
        tunnel: w137 -> [w183] mode=indexing
        n54 = call "String To Dbl.vi"("String"=w183) -> ("Numeric"=w182:dbl)  [unwired: 10 in]
        n55 = call "String To Dbl.vi"("String"=w191) -> ("Numeric"=w190:dbl)  [unwired: 10 in]
        n56 = call "String To Dbl.vi"("String"=w188) -> ("Numeric"=w189:dbl)  [unwired: 10 in]
        n57 = call "String To Dbl.vi"("String"=w184) -> ("Numeric"=w185:dbl)  [unwired: 10 in]
        n58 = call "String To Dbl.vi"("String"=w195) -> ("Numeric"=w194:dbl)  [unwired: 10 in]
        n59 = call "String To Dbl.vi"("String"=w193) -> ("Numeric"=w192:dbl)  [unwired: 10 in]
        n60 = call "String To Dbl.vi"("String"=w187) -> ("Numeric"=w186:dbl)  [unwired: 10 in]
      }
      n61 = Build Array(w115) -> (w129:dbl[])
      n62 = call <vilib>:"Interpolate 1D.vi"("method"=w128, "xi"=w129, "X"=w130, "Y"=w181) -> ("yi"=w180:dbl[])  [unwired: 5 in, 2 out]
      n63 = call <vilib>:"Interpolate 1D.vi"("method"=w128, "xi"=w129, "X"=w130, "Y"=w165) -> ("yi"=w163:dbl[])  [unwired: 5 in, 2 out]
      n64 = call <vilib>:"Interpolate 1D.vi"("method"=w128, "xi"=w129, "X"=w130, "Y"=w160) -> ("yi"=w162:dbl[])  [unwired: 5 in, 2 out]
      n65 = call <vilib>:"Interpolate 1D.vi"("method"=w128, "xi"=w129, "X"=w130, "Y"=w143) -> ("yi"=w145:dbl[])  [unwired: 5 in, 2 out]
      n66 = call <vilib>:"Interpolate 1D.vi"("method"=w128, "xi"=w129, "X"=w130, "Y"=w134) -> ("yi"=w133:dbl[])  [unwired: 5 in, 2 out]
      n67 = call <vilib>:"Interpolate 1D.vi"("method"=w128, "xi"=w129, "X"=w130, "Y"=w151) -> ("yi"=w149:dbl[])  [unwired: 5 in, 2 out]
      n68 = Index Array(array=w133) -> (element=w131:dbl)  [unwired: 1 in]
      n69 = Index Array(array=w180) -> (element=w179:dbl)  [unwired: 1 in]
      n70 = Index Array(array=w163) -> (element=w164:dbl)  [unwired: 1 in]
      n71 = Index Array(array=w162) -> (element=w161:dbl)  [unwired: 1 in]
      n72 = Index Array(array=w145) -> (element=w144:dbl)  [unwired: 1 in]
      n73 = Index Array(array=w149) -> (element=w150:dbl)  [unwired: 1 in]
      n74 = Random Number (0-1)() -> (number: 0 to 1=w108:dbl)
      n75 = Random Number (0-1)() -> (number: 0 to 1=w121:dbl)
      n76 = Random Number (0-1)() -> (number: 0 to 1=w113:dbl)
      n77 = Random Number (0-1)() -> (number: 0 to 1=w111:dbl)
      n78 = Divide(x=w108, y=50.0) -> (x/y=w106:dbl)
      n79 = Divide(x=w121, y=50.0) -> (x/y=w120:dbl)
      n80 = Divide(x=w113, y=150.0) -> (x/y=w112:dbl)
      n81 = Divide(x=w111, y=150.0) -> (x/y=w109:dbl)
      n82 = Add(x=w179, y=w106) -> (x+y=w116:dbl)
      n83 = Add(x=w106, y=w164) -> (x+y=w127:dbl)
      n84 = Add(x=w106, y=w144) -> (x+y=w124:dbl)
      n85 = Add(x=w131, y=w120) -> (x+y=w123:dbl)
      n86 = Add(x=w112, y=w161) -> (x+y=w126:dbl)
      n87 = Add(x=w150, y=w109) -> (x+y=w125:dbl)
      n88 = Add(x=w106, y=w103) -> (x+y=w104:dbl)
      n89 = Add(x=w115, y=w104) -> (x+y=w105:dbl)
    }
    frame "VUOTO" {
      w230 = 13  # index (col)
      w238 = 16  # eff
      w240 = 15  # p2
      w247 = 14  # P1
      w260 = 10  # I
      w220 = 1 items=["nearest", "linear", "spline", "cubic Hermite", "Lagrange"] ("method")
      w211 = 9  # V
      w210 = 2  # RPM
      n90 = Index Array(array="VUOTO", index (col) #1=w211, index (col) #2=w210, index (col) #3=w260, index (col) #4=w247, index (col) #5=w240, index (col) #6=w238, index (col) #7=w230) -> (element #1=w270:string[], element #2=w264:string[], element #3=w259:string[], element #4=w249:string[], element #5=w239:string[], element #6=w231:string[], element #7=w224:string[])  [unwired: 7 in]
      n91 = Delete From Array(array=w224, length=1, index=0) -> (array with subset deleted=w229:string[])  [unwired: 1 out]
      n92 = Delete From Array(array=w270, length=1, index=0) -> (array with subset deleted=w269:string[])  [unwired: 1 out]
      n93 = Delete From Array(array=w264, length=1, index=0) -> (array with subset deleted=w263:string[])  [unwired: 1 out]
      n94 = Delete From Array(array=w259, length=1, index=0) -> (array with subset deleted=w258:string[])  [unwired: 1 out]
      n95 = Delete From Array(array=w249, length=1, index=0) -> (array with subset deleted=w248:string[])  [unwired: 1 out]
      n96 = Delete From Array(array=w231, length=1, index=0) -> (array with subset deleted=w232:string[])  [unwired: 1 out]
      n97 = Delete From Array(array=w239, length=1, index=0) -> (array with subset deleted=w246:string[])  [unwired: 1 out]
      n98 = for {
        tunnel: w269 -> [w287] mode=indexing
        tunnel: [w286] -> w222 mode=indexing
        tunnel: w263 -> [w285] mode=indexing
        tunnel: [w284] -> w273 mode=indexing
        tunnel: w258 -> [w283] mode=indexing
        tunnel: [w282] -> w257 mode=indexing
        tunnel: [w281] -> w252 mode=indexing
        tunnel: w248 -> [w280] mode=indexing
        tunnel: [w278] -> w243 mode=indexing
        tunnel: w246 -> [w279] mode=indexing
        tunnel: [w277] -> w235 mode=indexing
        tunnel: w232 -> [w276] mode=indexing
        tunnel: [w274] -> w226 mode=indexing
        tunnel: w229 -> [w275] mode=indexing
        n99 = call "String To Dbl.vi"("String"=w275) -> ("Numeric"=w274:dbl)  [unwired: 10 in]
        n100 = call "String To Dbl.vi"("String"=w283) -> ("Numeric"=w282:dbl)  [unwired: 10 in]
        n101 = call "String To Dbl.vi"("String"=w280) -> ("Numeric"=w281:dbl)  [unwired: 10 in]
        n102 = call "String To Dbl.vi"("String"=w276) -> ("Numeric"=w277:dbl)  [unwired: 10 in]
        n103 = call "String To Dbl.vi"("String"=w287) -> ("Numeric"=w286:dbl)  [unwired: 10 in]
        n104 = call "String To Dbl.vi"("String"=w285) -> ("Numeric"=w284:dbl)  [unwired: 10 in]
        n105 = call "String To Dbl.vi"("String"=w279) -> ("Numeric"=w278:dbl)  [unwired: 10 in]
      }
      n106 = Build Array(w201) -> (w221:dbl[])
      n107 = call <vilib>:"Interpolate 1D.vi"("method"=w220, "xi"=w221, "X"=w222, "Y"=w273) -> ("yi"=w272:dbl[])  [unwired: 5 in, 2 out]
      n108 = call <vilib>:"Interpolate 1D.vi"("method"=w220, "xi"=w221, "X"=w222, "Y"=w257) -> ("yi"=w255:dbl[])  [unwired: 5 in, 2 out]
      n109 = call <vilib>:"Interpolate 1D.vi"("method"=w220, "xi"=w221, "X"=w222, "Y"=w252) -> ("yi"=w254:dbl[])  [unwired: 5 in, 2 out]
      n110 = call <vilib>:"Interpolate 1D.vi"("method"=w220, "xi"=w221, "X"=w222, "Y"=w235) -> ("yi"=w237:dbl[])  [unwired: 5 in, 2 out]
      n111 = call <vilib>:"Interpolate 1D.vi"("method"=w220, "xi"=w221, "X"=w222, "Y"=w226) -> ("yi"=w225:dbl[])  [unwired: 5 in, 2 out]
      n112 = call <vilib>:"Interpolate 1D.vi"("method"=w220, "xi"=w221, "X"=w222, "Y"=w243) -> ("yi"=w241:dbl[])  [unwired: 5 in, 2 out]
      n113 = Index Array(array=w225) -> (element=w223:dbl)  [unwired: 1 in]
      n114 = Index Array(array=w272) -> (element=w271:dbl)  [unwired: 1 in]
      n115 = Index Array(array=w255) -> (element=w256:dbl)  [unwired: 1 in]
      n116 = Index Array(array=w254) -> (element=w253:dbl)  [unwired: 1 in]
      n117 = Index Array(array=w237) -> (element=w236:dbl)  [unwired: 1 in]
      n118 = Index Array(array=w241) -> (element=w242:dbl)  [unwired: 1 in]
      n119 = Random Number (0-1)() -> (number: 0 to 1=w200:dbl)
      n120 = Divide(x=w200, y=50.0) -> (x/y=w198:dbl)
      n121 = Random Number (0-1)() -> (number: 0 to 1=w213:dbl)
      n122 = Random Number (0-1)() -> (number: 0 to 1=w207:dbl)
      n123 = Random Number (0-1)() -> (number: 0 to 1=w205:dbl)
      n124 = Divide(x=w213, y=50.0) -> (x/y=w212:dbl)
      n125 = Divide(x=w207, y=150.0) -> (x/y=w206:dbl)
      n126 = Divide(x=w205, y=150.0) -> (x/y=w203:dbl)
      n127 = Add(x=w198, y=w197) -> (x+y=w196:dbl)
      n128 = Add(x=w271, y=w198) -> (x+y=w209:dbl)
      n129 = Add(x=w198, y=w256) -> (x+y=w219:dbl)
      n130 = Add(x=w198, y=w236) -> (x+y=w216:dbl)
      n131 = Add(x=w223, y=w212) -> (x+y=w215:dbl)
      n132 = Add(x=w206, y=w253) -> (x+y=w218:dbl)
      n133 = Add(x=w242, y=w203) -> (x+y=w217:dbl)
    }
  }
  "C[nm]" <- w12
  "I[A]" <- w11
  "Pin kw" <- w10
  "Pout kw" <- w9
  "eff%" <- w8
  "cosfi" <- w7
  "RPM" <- w3
